vi "Get Pressure Module Idn.vi"(8 "error in (no error)":errorcluster, 11 "VISA resource name":refnum<visa-resource-name>) -> (0 "error out":errorcluster, 1 "Model Number":string, 2 "Manufacturer":string, 3 "VISA resource name out":refnum<visa-resource-name>, 4 "Serial Number":string)   [LabVIEW 2011, in "Fluke 5XXX Series Multicalibrators.lvlib"]
doc: "This VI queries the attached pressure module for its model and serial number.\n\nNote:\n\nThis VI is available only for instrument model 5520A with Fluke 700-Pxx external pressure modules."
uses:
  Fluke 5XXX Series Multicalibrators.lvlib
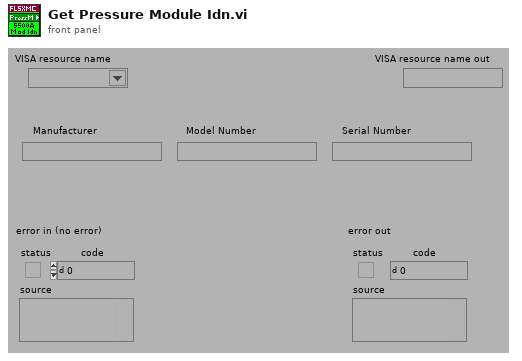
[diagram p1: front panel]
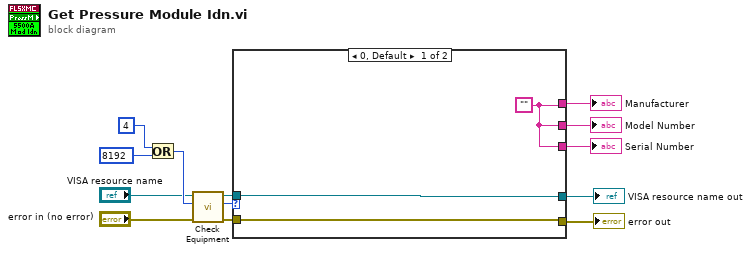
[diagram p0: block diagram]
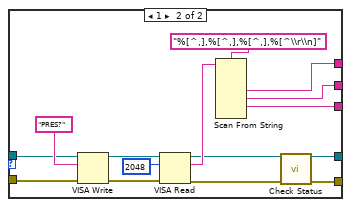
[diagram p2: hidden frame]
diagram:
  n1 = Or(x=4 ("Numeric"), y=8192 ("Numeric")) -> (x .or. y?=w9:i32)
  n2 = call "Check Equipment.vi"("error in (no error)"="error in (no error)", "Bit Mask"=w9, "VISA resource name"="VISA resource name") -> ("error out"=w13:errorcluster, "Present?"=w12:u32, "VISA resource name out"=w11:refnum<visa-resource-name>)  [unwired: 6 in]
  n3 = case shown="0, Default" w12 {
    tunnel: [w16 w21] -> w6
    tunnel: [w15 w20] -> w5
    tunnel: w13 -> [w16 w23]
    tunnel: w11 -> [w15 w22]
    tunnel: [w14 w19] -> w4
    tunnel: [w14 w18] -> w3
    tunnel: [w14 w17] -> w2
    frame 0, Default {
      w14 = ""
    }
    frame 1 {
      n4 = VISA Write(VISA resource name=w22, write buffer="PRES?", error in (no error)=w23) -> (VISA resource name out=w25:refnum<visa-resource-name>, error out=w26:errorcluster)  [unwired: 1 out]
      n5 = VISA Read(VISA resource name=w25, byte count=u32 2048 ("byte count (0)"), error in (no error)=w26) -> (VISA resource name out=w30:refnum<visa-resource-name>, read buffer=w31:string, error out=w29:errorcluster)  [unwired: 1 out]
      n6 = Scan From String(format string="%[^,],%[^,],%[^,],%[^\\r\\n]", input string=w31) -> (output 1=w19:string, output 2=w18:string, output 3=w17:string)  [unwired: 7 in, 3 out]
      n7 = call "Check Status.vi"("VISA resource name"=w30, "error in (no error)"=w29) -> ("VISA resource name out"=w20:refnum<visa-resource-name>, "error out"=w21:errorcluster)  [unwired: 12 in]
    }
  }
  "Manufacturer" <- w4
  "Model Number" <- w3
  "Serial Number" <- w2
  "VISA resource name out" <- w5
  "error out" <- w6
